vi "LJ_write_DB.vi"(2 "error in":errorcluster, 3 "Authentication":T3, 4 "database_ip":T1, 5 "Data to add":T2) -> (0 "error out":errorcluster)   [LabVIEW 2019]
uses:
  lv_mysql_connector_v1_lv8/typedefs/mysql_authentication.ctl
  Type defs/Database_control.ctl
  Type defs/cred_ip_info.ctl
panel:
  out "concatenated string":string
  in  "Port":u16=13306
  in  "IP Address":string="128.40.177.193"
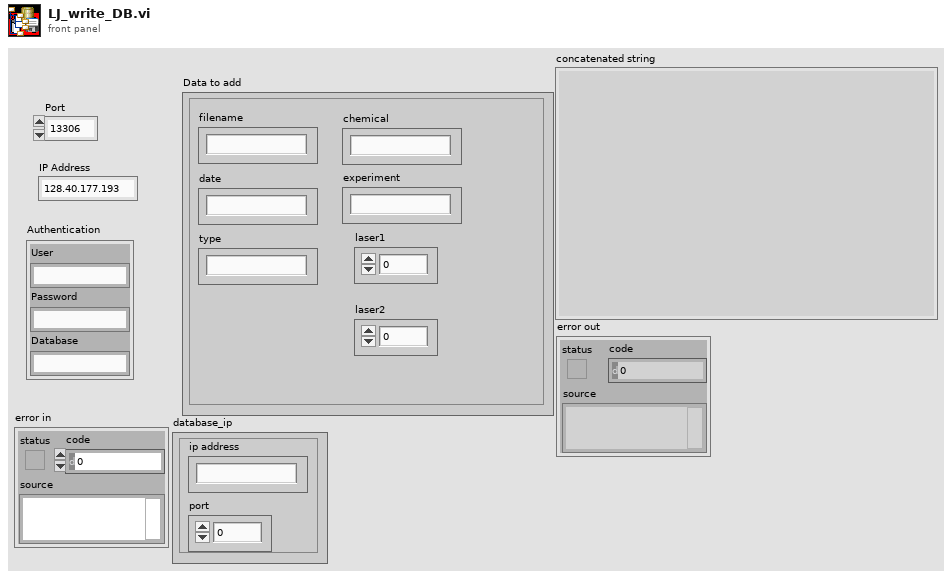
[diagram p1: front panel]
types:
  T1 = typedef "cred_ip_info.ctl" = cluster{"ip address":string, "port":dbl}
  T2 = typedef "Database_control.ctl" = cluster{"filename":string, "date":string, "type":string, "chemical":string, "experiment":string, "laser1":dbl, "laser2":dbl}
  T3 = typedef "mysql_authentication.ctl" = cluster{"User":string, "Password":string, "Database":string}
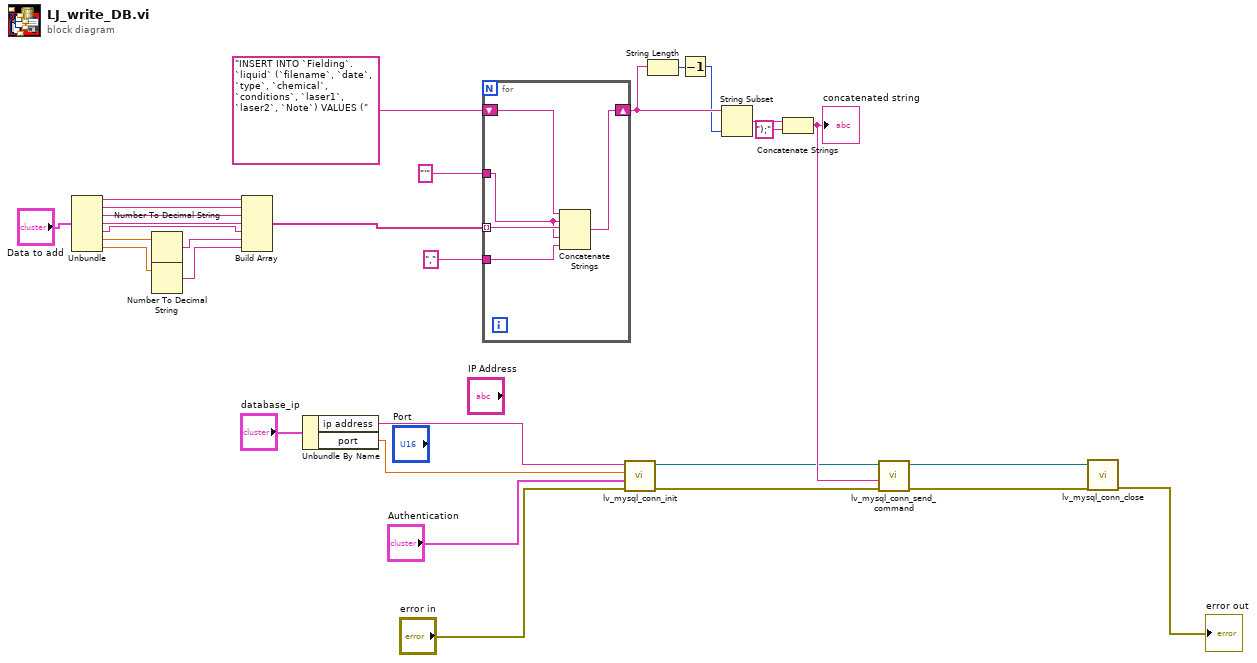
[diagram p0: block diagram]
diagram:
  n1 = Unbundle("Data to add") -> ("filename"=w27:string, "date"=w26:string, "type"=w25:string, "chemical"=w24:string, "experiment"=w23:string, "laser1"=w29:dbl, "laser2"=w28:dbl)
  n2 = Number To Decimal String(number=w29) -> (decimal integer string=w22:string)  [unwired: 1 in]
  n3 = Number To Decimal String(number=w28) -> (decimal integer string=w21:string)  [unwired: 1 in]
  n4 = Build Array(w27, w26, w25, w24, w23, w22, w21) -> (w20:string[])
  n5 = Unbundle By Name("database_ip") -> ("ip address"=w2:string, "port"=w1:dbl)
  n6 = for {
    tunnel: w20 -> [w35] mode=indexing
    shift-right: [w31] -> w15
    shift-left: "INSERT INTO `Fielding`.`liquid` (`filename`, `date`, `type`, `chemical`, `conditions`, `laser1`, `laser2`, `Note`) VALUES (" -> [w34]
    tunnel: "'" ("string") -> [w33]
    tunnel: "," ("string") -> [w32]
    n7 = Concatenate Strings(w34, w33, w35, w33, w32) -> (w31:string)
  }
  n8 = call "lv_mysql_conn_init.vi"("error in (no error)"="error in", "Authentication"="Authentication", "Port"=w1, "IP Address"=w2) -> ("error out"=w7:errorcluster, "connection ID out"=w5:refnum<k5>)  [unwired: 6 in]
  n9 = String Length(string=w15) -> (length=w12:i32)
  n10 = Decrement(x=w12) -> (x-1=w13:i32)
  n11 = String Subset(string=w15, length (rest)=w13) -> (substring=w14:string)  [unwired: 1 in]
  n12 = Concatenate Strings(w14, ");" ("string")) -> (w11:string)
  "concatenated string" <- w11
  n13 = call "lv_mysql_conn_send_command.vi"("error in (no error)"=w7, "Message"=w11, "connection ID"=w5) -> ("error out"=w6:errorcluster, "connection ID out"=w4:refnum<k5>)  [unwired: 7 in]
  n14 = call "lv_mysql_conn_close.vi"("error in (no error)"=w6, "connection ID"=w4) -> ("error out"=→"error out":errorcluster)  [unwired: 9 in]
